vi "update.plot.vi"(8 "error in (no error)":errorcluster, 11 "manager_daemon in":refnum<class "manager_daemon.lvclass">) -> (0 "error out":errorcluster, 3 "manager_daemon out":refnum<class "manager_daemon.lvclass">)   [LabVIEW 2024, in "manager_daemon.lvclass"]
uses:
  manager_daemon.lvclass
  manager_daemon.lvclass/manager_daemon.ctl
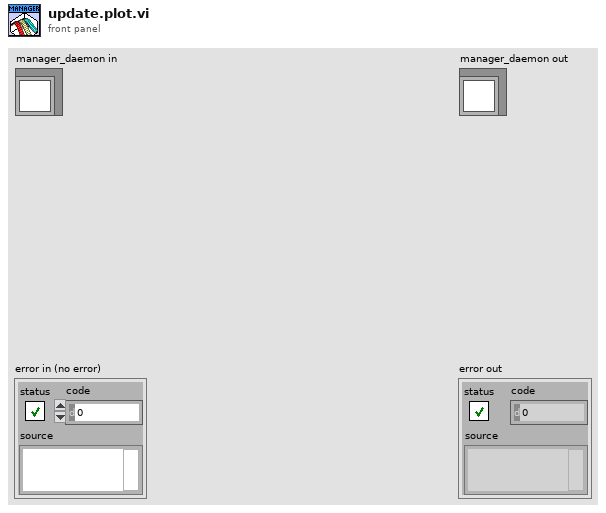
[diagram p1: front panel]
types:
  T1 = typedef "volume.object--cluster.ctl" = cluster{"start date":timestamp, "end date":timestamp, "sortable_name":string, "color":u32, "volume type":T2, "issues":T3[]}
  T2 = typedef "volume.type--enum.ctl" = enum16{"Ongoing", "Limited Series", "Annual", "One Shot", "Reprint/Document", "Star Comics", "Epic Comics"}
  T3 = typedef "issue.display--cluster.ctl" = cluster{"cover_date":timestamp, "id":i32, "number":string, "fill":bool}
  T4 = cluster{"filtered data":T1[], "filter dates":cluster{"start":timestamp, "end":timestamp}}
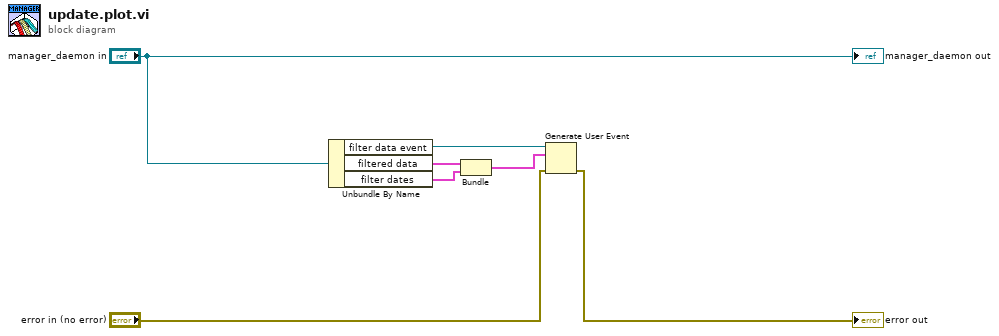
[diagram p0: block diagram]
diagram:
  n1 = Unbundle By Name("manager_daemon in") -> ("filter data event"=w7:refnum<user-event>, "filtered data"=w3:T1[], "filter dates"=w2:cluster{"start":timestamp, "end":timestamp})
  n2 = Bundle("filtered data"=w3, "filter dates"=w2) -> (w1:T4)  [unwired: 1 in]
  n3 = Generate User Event(user event=w7, event data cluster=w1, error in="error in (no error)") -> (error out=→"error out":errorcluster)  [unwired: 1 in, 1 out]
  "manager_daemon out" <- "manager_daemon in"
